vi "findFile.vi"(8 "Error In":errorcluster, 9 "Files":refnum<k24>[](array[refnum]), 10 "File Name":string) -> (0 "error out":errorcluster, 2 "File Reference":refnum<k24>)   [LabVIEW 2016, in "GDrive.lvlib"]
doc: "This VI is designed to output a reference to a specific file, given that file's name."
uses:
  GDrive.lvlib
  C:/Users/motoole/Desktop/VC OToolekit/Dependencies/Google.Apis.Drive.v3.dll
  Dependencies/Google.Apis.Drive.v3.dll
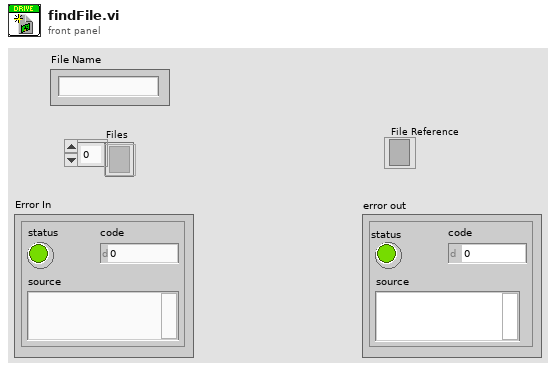
[diagram p1: front panel]
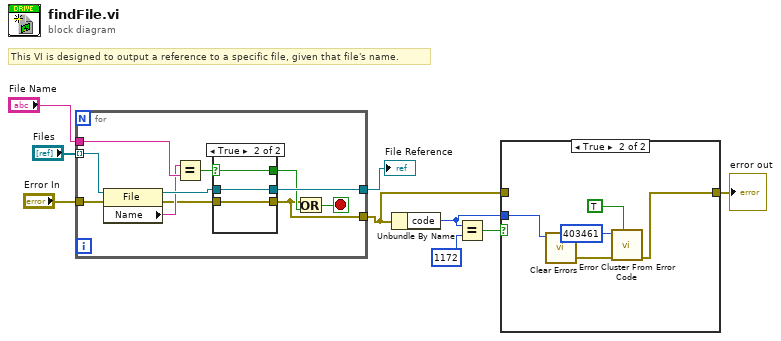
[diagram p0: block diagram]
diagram:
  # "This VI is designed to output a reference to a specific file, given that file's name."
  n1 = for {
    tunnel: "Files" -> [w20] mode=indexing
    tunnel: "File Name" -> [w19]
    tunnel: [w18] -> w7
    tunnel: "Error In" -> [w16]
    tunnel: [w10] -> w3
    stop <- w12 stop-if-true
    n2 = property class="File"(reference=w20, error in=w16) -> (reference out=w17:refnum<k24>, error out=w13:errorcluster, "Name"=w14:string)
    n3 = Equal?(x=w14, y=w19) -> (x = y?=w15:bool)
    n4 = case shown="True" w15 {
      selector: w15 -> [w21 w23]
      tunnel: [_ w25] -> w18
      tunnel: w17 -> [_ w25]
      tunnel: [w22 w24] -> w10
      tunnel: w13 -> [w22 w24]
      tunnel: [w21 w23] -> w11
      frame False {
      }
      frame True {
      }
    }
    n5 = Or(x=w10, y=w11) -> (x .or. y?=w12:bool)
  }
  "File Reference" <- w7
  n6 = Unbundle By Name(w3) -> ("code"=w1:i32)
  n7 = Equal?(x=w1, y=1172) -> (x = y?=w4:bool)
  n8 = case shown="True" w4 {
    tunnel: w3 -> [w26 _]
    tunnel: [w26 w31] -> w2
    tunnel: w1 -> [_ w29]
    frame False {
    }
    frame True {
      n9 = call <vilib>:"Clear Errors.vi"("specific error code to clear (0: all)"=w29) -> ("error out"=w30:errorcluster)  [unwired: 5 in, 1 out]
      n10 = call <vilib>:"Error Cluster From Error Code.vi"("show call chain? (False)"=TRUE, "error in (no error)"=w30, "error code (0)"=403461) -> ("error out"=w31:errorcluster)  [unwired: 6 in]
    }
  }
  "error out" <- w2
